vi "Append Digit.vi"(1 "New Char":string, 2 "Existing String":string) -> (0 "Resulting String":string)   [LabVIEW 2014]
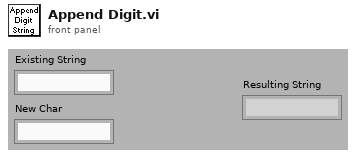
[diagram p1: front panel]
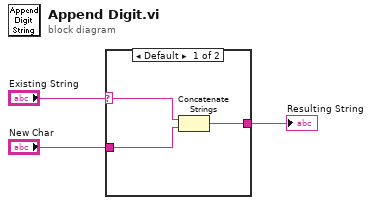
[diagram p0: block diagram]
diagram:
  n1 = case shown="Default" "Existing String" {
    selector: "Existing String" -> [w6 _]
    tunnel: "New Char" -> [w5 w7]
    tunnel: [w4 w7] -> w1
    frame Default {
      n2 = Concatenate Strings(w6, w5) -> (w4:string)
    }
    frame "0" {
    }
  }
  "Resulting String" <- w1
